vi "DependencyViewer Main.vi"(10 "Object":u64, 11 "Sub Command":string) -> ()   [LabVIEW 2020]
uses:
  <vilib>/Utility/sysdir.llb/System Directory Type.ctl
  <resource>/Framework/Providers/Open_GDS/DependencyViewer/DependencyChecker/DependencyChecker.lvlib
  <resource>/Framework/Providers/Open_GDS/DependencyViewer/VISJS-Viewer/VISJS Viewer.lvlib
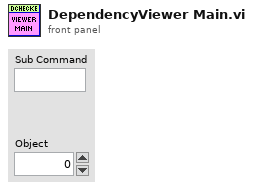
[diagram p1: front panel]
types:
  T1 = typedef "GOOP_DependencySettings.ctl" = cluster{"EmbedChartLibraryScript":bool, "Configurations":T2[], "UseProjectFolder":bool, "Folder to save reports to":path, "Max reports to save":u8}
  T2 = typedef "DependencyChecker.lvlib/DependencyConfiguration.ctl" = cluster{"Name":string, "RemoveItemsBelongingToLibraries":bool, "RemoveEvenSubLibraries":bool, "FilterOptions":T3, "OnlyKeepCircularDepedencies":bool, "IgnoreLibrariesInCircularDependencies":bool}
  T3 = typedef "DependencyChecker.lvlib/FilterOptions.ctl" = cluster{"Ignore user.lib":bool, "Ignore vi.lib":bool, "Ignore instr.lib":bool, "FolderToIgnore":path[], "Ignore libraries":bool, "Ignore lvcasses":bool, "Ignore xnodes":bool, "Ignore xcontrols":bool, "Ignore Channel Classes":bool}
  T4 = typedef "DependencyChecker.lvlib/LibraryDependentInfo.vi" = cluster{"Type":T5, "Path":path, "FullQualifierName":string, "DependentLibrary":map{path, set{path}}, "ParentLibraries":path[], "IsInterface":bool}
  T5 = typedef "NI_FileType.lvlib/FT_FileTypes.ctl" = enum32{"Invalid file/path", "Unknown type", "Instrument", "Control", "Polymorphic VI", "Project", "Library", "LVClass", "XControl", "XNode", "CIN", "Run-time menu", "Palette menu", "LLB", "Shortcut", "Directory", "Class Private Data Control", "Statechart", "MathScript .m file", "Ladder Diagram", "LVLibp"}
  T6 = typedef "DependencyChecker.lvlib/FileDependencyType.ctl" = cluster{"Path":path, "FileType":T5, "FullQualifierName":string, "OwnerPath":path, "Dependencies":path[], "ParentLibraries":path[], "IsInterface":bool}
  T7 = typedef "System Directory Type.ctl" = i32
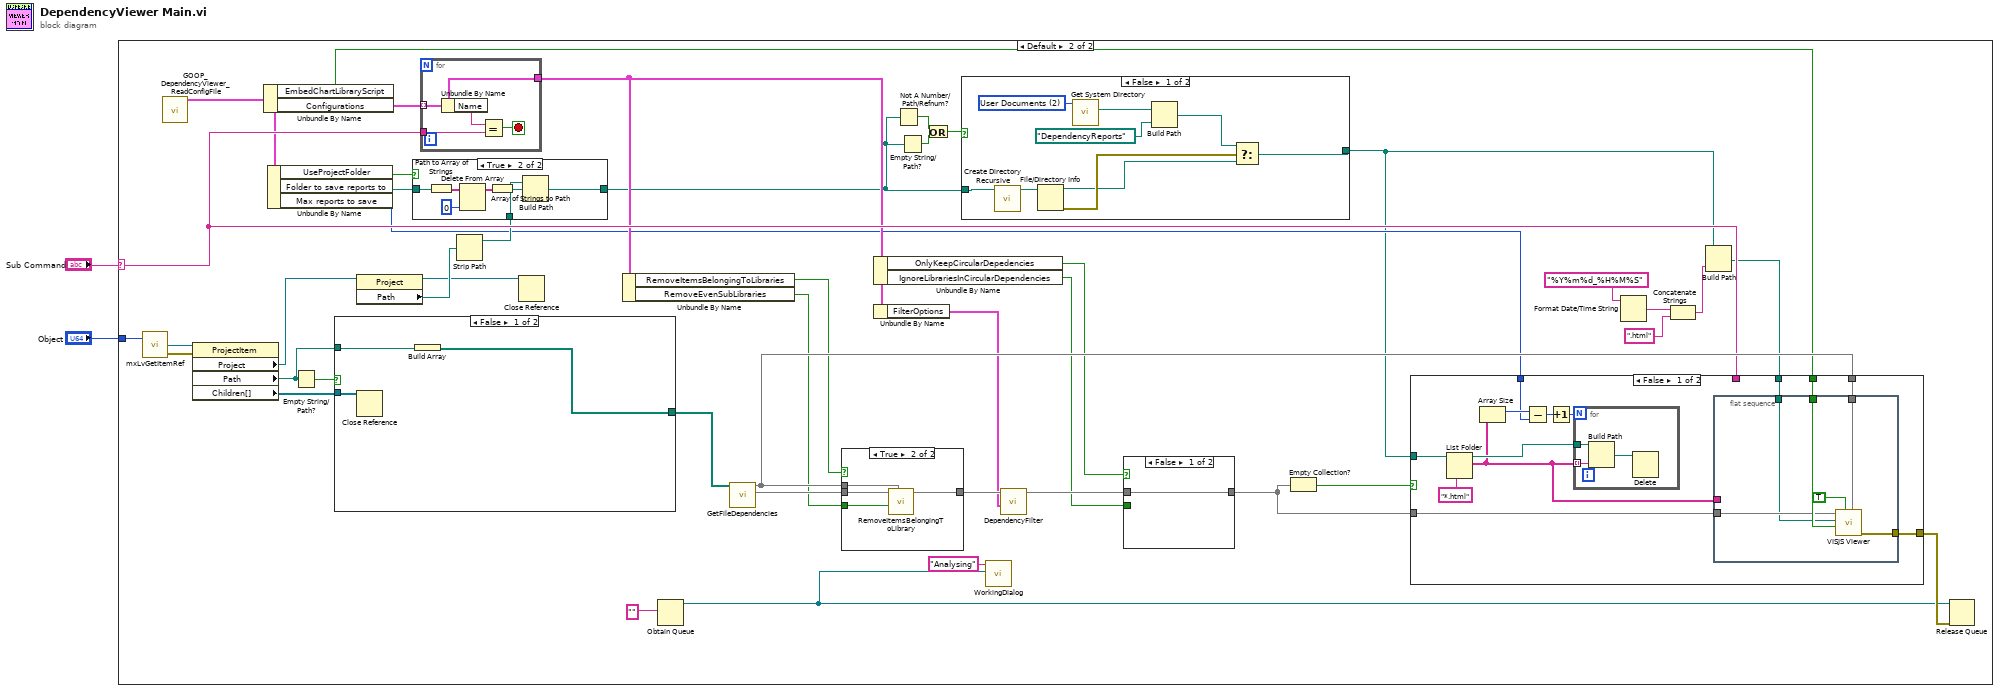
[diagram p0: block diagram]
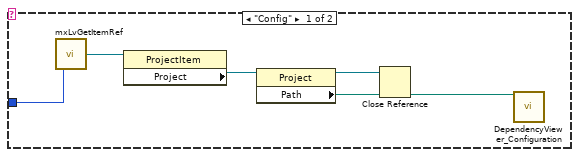
[diagram p2: hidden frame]
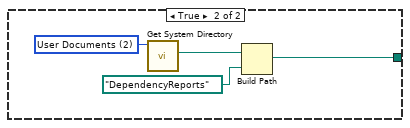
[diagram p3: hidden frame]
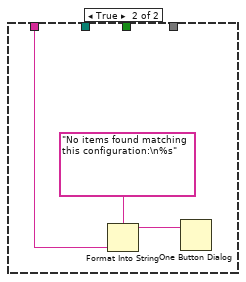
[diagram p5: hidden frame]
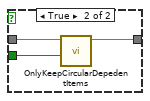
[diagram p6: hidden frame]
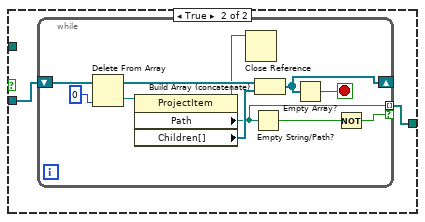
[diagram p7: hidden frame]
diagram:
  n1 = case shown="Default" "Sub Command" {
    selector: "Sub Command" -> [_ w31]
    tunnel: "Object" -> [w7 w49]
    frame "Config" {
      n2 = call <resource>:"mxLvGetItemRef.vi"("Item"=w7) -> ("Item Refnum"=w6:refnum<vi>)  [unwired: 1 in, 2 out]
      n3 = property class="ProjectItem"(reference=w6) -> ("Project"=w5:refnum<vi>)  [unwired: 1 in, 2 out]
      n4 = property class="Project"(reference=w5) -> (reference out=w4:refnum<vi>, "Path"=w3:path)  [unwired: 1 in, 1 out]
      n5 = Close Reference(reference=w4) -> ()  [unwired: 1 in, 1 out]
      n6 = call <resource>:"DependencyViewer_Configuration.vi"("ProjectPath"=w3) -> ()  [unwired: 10 in, 1 out]
    }
    frame Default {
      n7 = call <resource>:"mxLvGetItemRef.vi"("Item"=w49) -> ("Item Refnum"=w51:refnum<vi>, "error out"=w50:errorcluster)  [unwired: 1 in, 1 out]
      n8 = call <resource>:"GOOP_DependencyViewer_ReadConfigFile.vi"() -> ("Config"=w29:T1)  [unwired: 11 in]
      n9 = property class="ProjectItem"(reference=w51, error in=w50) -> ("Project"=w26:refnum<vi>, "Path"=w34:path, "Children[]"=w37:refnum<vi>[])  [unwired: 2 out]
      n10 = Unbundle By Name(w29) -> ("EmbedChartLibraryScript"=w38:bool, "Configurations"=w44:T2[])
      n11 = Unbundle By Name(w29) -> ("UseProjectFolder"=w28:bool, "Folder to save reports to"=w27:path, "Max reports to save"=w17:u8)
      n12 = Empty String/Path?(string/path=w34) -> (empty?=w35:bool)
      n13 = case shown="False" w35 {
        tunnel: w37 -> [w102 w106]
        tunnel: [w103 w105] -> w36
        tunnel: w34 -> [w104 _]
        frame False {
          n14 = Close Reference(reference=w102) -> ()  [unwired: 1 in, 1 out]
          n15 = Build Array(w104) -> (w103:path[])
        }
        frame True {
          n16 = while {
            shift-right: [w112] -> _
            shift-left: w106 -> [w117]
            tunnel: [w110] -> w105 mode=indexing if=w108
            stop <- w111 stop-if-true
            n17 = Delete From Array(array=w117, index=0) -> (deleted portion=w115:refnum<vi>, array with subset deleted=w114:refnum<vi>[])  [unwired: 1 in]
            n18 = property class="ProjectItem"(reference=w115) -> (reference out=w107:refnum<vi>, "Path"=w110:path, "Children[]"=w113:refnum<vi>[])  [unwired: 1 in, 1 out]
            n19 = Close Reference(reference=w107) -> ()  [unwired: 1 in, 1 out]
            n20 = Empty String/Path?(string/path=w110) -> (empty?=w109:bool)
            n21 = Build Array (concatenate)(w114, w113) -> (w112:refnum<vi>[])
            n22 = Empty Array?(array=w112) -> (empty?=w111:bool)
            n23 = Not(x=w109) -> (.not. x?=w108:bool)
          }
        }
      }
      n24 = property class="Project"(reference=w26) -> (reference out=w24:refnum<vi>, "Path"=w25:path)  [unwired: 1 in, 1 out]
      n25 = for {
        tunnel: w44 -> [w123] mode=indexing
        tunnel: w31 -> [w125]
        tunnel: [w123] -> w30
        stop <- w124 stop-if-true
        n26 = Unbundle By Name(w123) -> ("Name"=w126:string)
        n27 = Equal?(x=w126, y=w125) -> (x = y?=w124:bool)
      }
      n28 = Strip Path(path=w25) -> (stripped path=w23:path)  [unwired: 1 out]
      n29 = case shown="True" w28 {
        tunnel: w27 -> [w65 w71]
        tunnel: w23 -> [_ w72]
        tunnel: [w65 w66] -> w15
        frame False {
        }
        frame True {
          n30 = Path to Array of Strings(0:w71) -> (2:w70:string[])  [unwired: 1 out]
          n31 = Delete From Array(array=w70, index=0) -> (array with subset deleted=w68:string[])  [unwired: 1 in, 1 out]
          n32 = Array of Strings to Path(0:w68) -> (2:w67:path)  [unwired: 1 in]
          n33 = Build Path(base path=w72, name or relative path=w67) -> (appended path=w66:path)
        }
      }
      n34 = Close Reference(reference=w24) -> ()  [unwired: 1 in, 1 out]
      n35 = Unbundle By Name(w30) -> ("RemoveItemsBelongingToLibraries"=w43:bool, "RemoveEvenSubLibraries"=w42:bool)
      n36 = Obtain Queue(element data type="") -> (queue out=w8:refnum<queue>)  [unwired: 4 in, 2 out]
      n37 = call <resource>:"GetFileDependencies.vi"("All Files in Dir"=w36) -> ("LibraryDependency"=w45:map{path, T4}, "FileDependency out"=w48:map{path, T6})  [unwired: 9 in]
      n38 = case shown="True" w43 {
        tunnel: w48 -> [_ w122]
        tunnel: [w118 w121] -> w46
        tunnel: w45 -> [w118 w120]
        tunnel: w42 -> [_ w119]
        frame False {
        }
        frame True {
          n39 = call <resource>:"RemoveItemsBelongingToLibrary.vi"("FileDependency In"=w122, "EvenSubLibraries"=w119, "LibraryDependency In"=w120) -> ("LibraryDependency Out"=w121:map{path, T4})  [unwired: 8 in]
        }
      }
      n40 = Unbundle By Name(w30) -> ("OnlyKeepCircularDepedencies"=w40:bool, "IgnoreLibrariesInCircularDependencies"=w39:bool)
      n41 = Unbundle By Name(w30) -> ("FilterOptions"=w41:T3)
      n42 = Not A Number/Path/Refnum?(number/path/refnum=w15) -> (NaN/Path/Refnum?=w14:bool)
      n43 = Empty String/Path?(string/path=w15) -> (empty?=w13:bool)
      n44 = Or(x=w14, y=w13) -> (x .or. y?=w12:bool)
      n45 = case shown="False" w12 {
        tunnel: [w56 w61] -> w16
        tunnel: w15 -> [w60 _]
        frame False {
          w53 = T7 2 items=["User Home"=0, "User Desktop"=1, "User Documents"=2, "User Application Data"=3, "User Preferences"=4, "User Temporary"=5, "Public Documents"=6, "Public Application Data"=7, "Public Preferences"=8, "Public Cache"=13, "System Core Libraries"=9, "System Installed Libraries"=10, "Application Files"=11, "Boot Volume Root"=12] ("system directory type")
          n46 = call <vilib>:"Create Directory Recursive.vi"("directory"=w60) -> ("directory copy"=w59:path)  [unwired: 4 in, 2 out]
          n47 = File/Directory Info(path=w59) -> (path out=w57:path, error out=w58:errorcluster)  [unwired: 1 in, 5 out]
          n48 = call <vilib>:"Get System Directory.vi"("system directory type"=w53) -> ("system directory"=w55:path)  [unwired: 10 in]
          n49 = Build Path(base path=w55, name or relative path=path "DependencyReports") -> (appended path=w52:path)
          n50 = Select(t=w52, s=w58, f=w57) -> (s? t:f=w56:path)
        }
        frame True {
          w62 = T7 2 items=["User Home"=0, "User Desktop"=1, "User Documents"=2, "User Application Data"=3, "User Preferences"=4, "User Temporary"=5, "Public Documents"=6, "Public Application Data"=7, "Public Preferences"=8, "Public Cache"=13, "System Core Libraries"=9, "System Installed Libraries"=10, "Application Files"=11, "Boot Volume Root"=12] ("system directory type")
          n51 = call <vilib>:"Get System Directory.vi"("system directory type"=w62) -> ("system directory"=w64:path)  [unwired: 10 in]
          n52 = Build Path(base path=w64, name or relative path=path "DependencyReports") -> (appended path=w61:path)
        }
      }
      n53 = call <resource>:"WorkingDialog.vi"("StopQueue"=w8, "Text"="Analysing") -> ()  [unwired: 10 in]
      n54 = call <resource>:"DependencyFilter.vi"("FilterOptions"=w41, "LibraryDependency In"=w46) -> ("Filtered LibraryDependency Out"=w47:map{path, T4})  [unwired: 9 in]
      n55 = case shown="False" w40 {
        tunnel: [w98 w101] -> w33
        tunnel: w47 -> [w98 w100]
        tunnel: w39 -> [_ w99]
        frame False {
        }
        frame True {
          n56 = call <resource>:"OnlyKeepCircularDepedentItems.vi"("IgnoreLibrariesInCircularDependencies(True)"=w99, "LibraryDependency In"=w100) -> ("LibraryDependency Out"=w101:map{path, T4})  [unwired: 9 in]
        }
      }
      n57 = Empty Collection?(1:w33) -> (0:w32:bool)
      n58 = Format Date/Time String(time format string (%c)="%Y%m%d_%H%M%S") -> (date/time string=w21:string)  [unwired: 2 in]
      n59 = Concatenate Strings(w21, ".html" ("string")) -> (w19:string)
      n60 = Build Path(base path=w16, name or relative path=w19) -> (appended path=w18:path)
      n61 = case shown="False" w32 {
        tunnel: w48 -> [w85 _]
        tunnel: w38 -> [w84 _]
        tunnel: w33 -> [w83 _]
        tunnel: w31 -> [_ w95]
        tunnel: w18 -> [w82 _]
        tunnel: w16 -> [w81 _]
        tunnel: w17 -> [w77 _]
        tunnel: [w74 _] -> w9
        frame False {
          n62 = List Folder(path=w81, pattern="*.html" ("string")) -> (path out=w79:path, filenames=w75:string[])  [unwired: 2 in, 2 out]
          n63 = Array Size(array=w75) -> (size(s)=w78:i32)
          n64 = Subtract(x=w78, y=w77) -> (x-y=w76:i32)
          n65 = Increment(x=w76) -> (x+1=w73:i32)
          n66 = for {
            N: w73 -> [_]
            tunnel: w75 -> [w93] mode=indexing
            tunnel: w79 -> [w94]
            n67 = Build Path(base path=w94, name or relative path=w93) -> (appended path=w92:path)
            n68 = Delete(path (use dialog)=w92) -> ()  [unwired: 4 in, 3 out]
          }
          n69 = flat-sequence {
            tunnel: w85 -> [w91]
            tunnel: w84 -> [w89]
            tunnel: w83 -> [w88]
            tunnel: w82 -> [w87]
            tunnel: w75 -> [_]
            tunnel: [w86] -> w74
            frame #0 {
              n70 = call <resource>:"VISJS Viewer.vi"("FileDependency In"=w91, "OpenWebBrowser(False)"=TRUE, "Embedd VISJS Librarya in HTMl File(False)"=w89, "HTMLFilePath"=w87, "LibraryDependency"=w88) -> ("error out"=w86:errorcluster)  [unwired: 5 in, 1 out]
            }
          }
        }
        frame True {
          n71 = Format Into String(format string="No items found matching this configuration:\n%s" ("message"), w95) -> (resulting string=w96:string)  [unwired: 2 in, 1 out]
          n72 = One Button Dialog(message=w96) -> ()  [unwired: 1 in, 1 out]
        }
      }
      n73 = Release Queue(queue=w8, error in (no error)=w9) -> ()  [unwired: 1 in, 3 out]
    }
  }
